vi "CreateNewSystemDefinition.vi"(7 "test VI ref":refnum<vi>, 8 "error in":errorcluster, 10 "OS (Windows)":string="Windows", 11 "System Definition Name":string) -> (0 "error out":errorcluster, 3 "System Definition Path":path)   [LabVIEW 2027, in "VeriStandTestUtilities.lvlib"]
uses:
  VeriStandTestUtilities.lvlib
  C:/NetCoreDLL/NationalInstruments.VeriStand.SystemDefinitionAPI.dll
  NetCoreDLL/NationalInstruments.VeriStand.SystemDefinitionAPI.dll
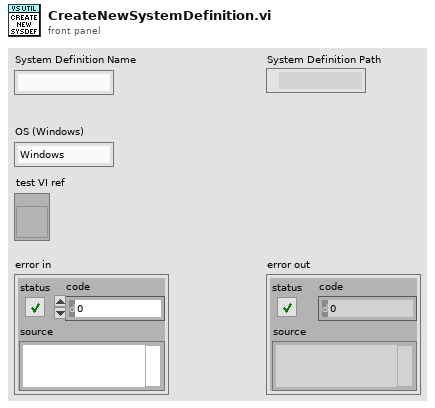
[diagram p1: front panel]
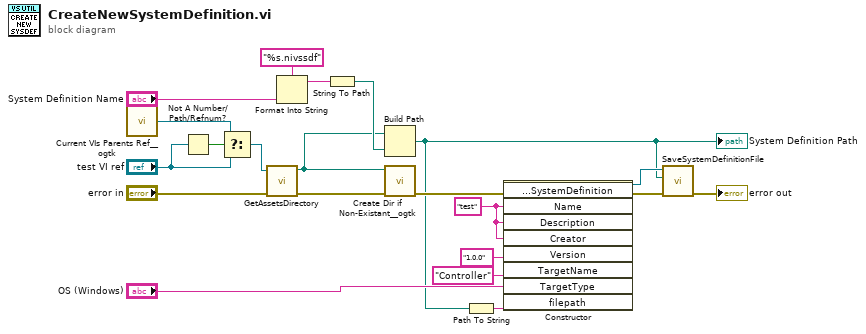
[diagram p0: block diagram]
diagram:
  w17 = "test" ("Name")
  n1 = call <userlib>:"Current VIs Parents Ref__ogtk.vi"() -> ("Calling VI's Reference"=w4:refnum<vi>)  [unwired: 2 in]
  n2 = Not A Number/Path/Refnum?(number/path/refnum="test VI ref") -> (NaN/Path/Refnum?=w1:bool)
  n3 = Select(t=w4, s=w1, f="test VI ref") -> (s? t:f=w3:refnum<vi>)
  n4 = call "GetAssetsDirectory.vi"("error in"="error in", "test VI refnum"=w3) -> ("error out"=w9:errorcluster, "assets dir"=w8:path)  [unwired: 8 in]
  n5 = Format Into String(format string="%s.nivssdf", "System Definition Name") -> (resulting string=w5:string)  [unwired: 2 in, 1 out]
  n6 = String To Path(string=w5) -> (path=w19:path)
  n7 = Build Path(base path=w8, name or relative path=w19) -> (appended path=w11:path)
  "System Definition Path" <- w11
  n8 = call <userlib>:"Create Dir if Non-Existant__ogtk.vi"("error in (no error)"=w9, "Directory Path"=w8) -> ("error out"=w18:errorcluster)  [unwired: 7 in, 2 out]
  n9 = Path To String(path=w11) -> (string=w13:string)
  n10 = constructor class="SystemDefinition"(error in=w18, "Name"=w17, "Description"=w17, "Creator"=w17, "Version"="1.0.0", "TargetName"="Controller", "TargetType"="OS (Windows)", "filepath"=w13) -> (reference out=w12:refnum<k39>, error out=w21:errorcluster)  [unwired: 2 in, 8 out]
  n11 = call "SaveSystemDefinitionFile.vi"("error in (no error)"=w21, "System Definition File in"=w11, "NationalInstruments.VeriStand.SystemDefinitionAPI.SystemDefinition"=w12) -> ("error out"=→"error out":errorcluster)  [unwired: 7 in, 1 out]
